vi "Configure Function.vi"(0 "VISA resource name":refnum<visa-resource-name>, 1 "Channel":i8 min=0 max=20 step=1, 5 "Function (5: Temp)":u16(ring)=5 items=["OFF", "VDC", "VAC", "OHMS", "FREQ", "TEMP"], 7 "Thermocouple Type (0: J) 2":u16(ring)=5 items=["J", "K", "E", "T", "N", "R", "S", "B", "C"], 9 "Frequency (0: 900 Hz)":u16(ring)=5 items=["900 Hz", "9 kHz", "90 kHz", "900 kHz", "1 MHz"], 11 "error in (no error)":errorcluster, 12 "Resistance (0: 300 Ohms)  2":u16(ring)=5 items=["300 Ohms", "3 k Ohms", "30 k Ohms", "300 k Ohms", "3 M Ohms", "10 M Ohms"], 13 "Voltage (0: 300 mV)  3":u16(ring)=5 items=["300 mV", "3 V", "30 V", "150/300 V", "3 M Ohms", "10 M Ohms"]) -> (4 "VISA resource name out":refnum<visa-resource-name>, 6 "concatenated string":string, 10 "read buffer":string, 15 "error out":errorcluster)   [LabVIEW 2013]
doc: "Configures the measurement type, resolution, and range on the instrument."
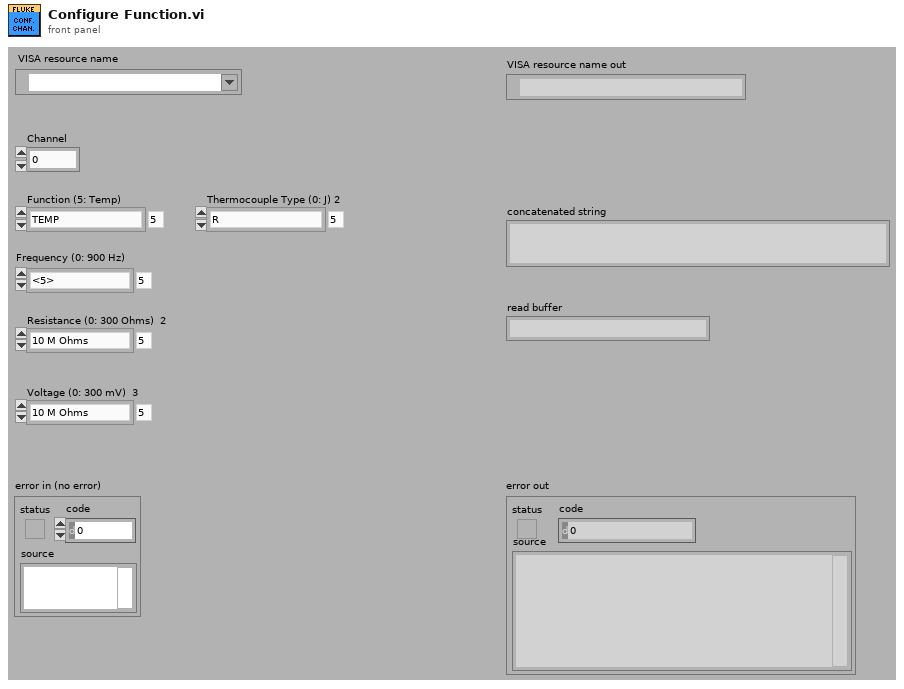
[diagram p1: front panel]
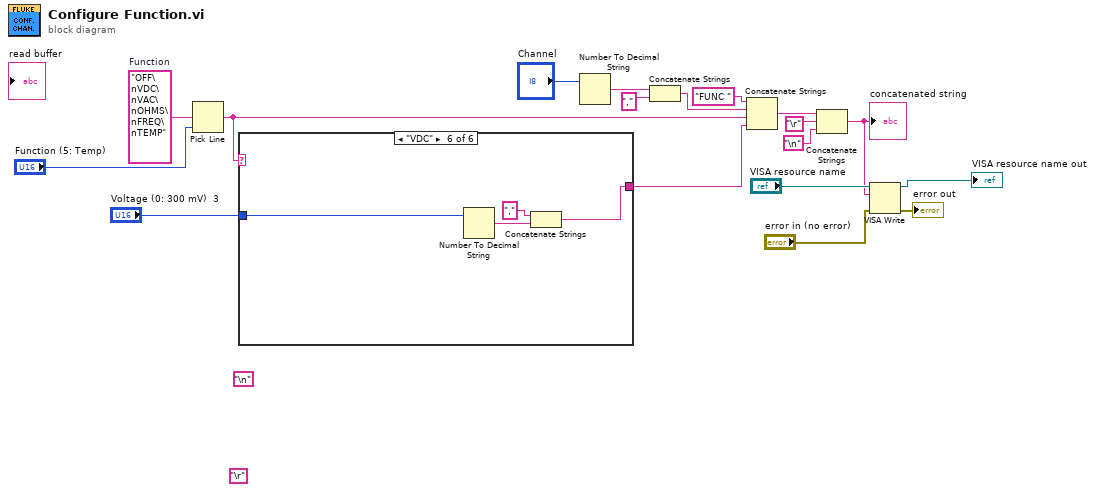
[diagram p0: block diagram]
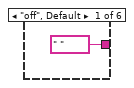
[diagram p2: hidden frame]
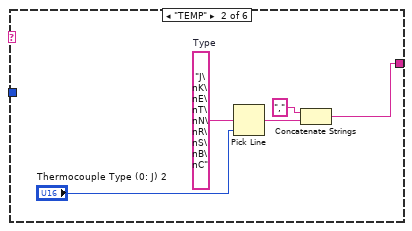
[diagram p3: hidden frame]
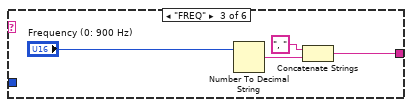
[diagram p4: hidden frame]
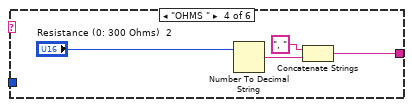
[diagram p5: hidden frame]
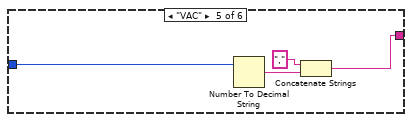
[diagram p6: hidden frame]
diagram:
  w18 = "OFF\nVDC\nVAC\nOHMS\nFREQ\nTEMP"  # Function
  (unwired) "\n"
  (unwired) "\r"
  n1 = Pick Line(multi-line string=w18, line index="Function (5: Temp)") -> (output string=w10:string)  [unwired: 1 in]
  n2 = case shown="\"VDC\"" w10 {
    tunnel: [" " w24 w27 w31 w33 w39] -> w11
    tunnel: "Voltage (0: 300 mV)  3" -> [_ _ _ _ w36 w40]
    frame "off", Default {
    }
    frame "TEMP" {
      w23 = "J\nK\nE\nT\nN\nR\nS\nB\nC"  # Type
      n3 = Pick Line(multi-line string=w23, line index="Thermocouple Type (0: J) 2") -> (output string=w21:string)  [unwired: 1 in]
      n4 = Concatenate Strings("," ("string"), w21) -> (w24:string)
    }
    frame "FREQ" {
      n5 = Number To Decimal String(number="Frequency (0: 900 Hz)") -> (decimal integer string=w25:string)  [unwired: 1 in]
      n6 = Concatenate Strings(", ", w25) -> (w27:string)
    }
    frame "OHMS " {
      n7 = Number To Decimal String(number="Resistance (0: 300 Ohms)  2") -> (decimal integer string=w29:string)  [unwired: 1 in]
      n8 = Concatenate Strings(", ", w29) -> (w31:string)
    }
    frame "VAC" {
      n9 = Number To Decimal String(number=w36) -> (decimal integer string=w34:string)  [unwired: 1 in]
      n10 = Concatenate Strings(",", w34) -> (w33:string)
    }
    frame "VDC" {
      n11 = Number To Decimal String(number=w40) -> (decimal integer string=w37:string)  [unwired: 1 in]
      n12 = Concatenate Strings(",", w37) -> (w39:string)
    }
  }
  n13 = Number To Decimal String(number="Channel") -> (decimal integer string=w14:string)  [unwired: 1 in]
  n14 = Concatenate Strings(w14, ",") -> (w12:string)
  n15 = Concatenate Strings("FUNC ", w12, w10, w11) -> (w6:string)
  n16 = Concatenate Strings(w6, "\r", "\n") -> (w2:string)
  "concatenated string" <- w2
  n17 = VISA Write(VISA resource name="VISA resource name", write buffer=w2, error in (no error)="error in (no error)") -> (VISA resource name out=→"VISA resource name out":refnum<visa-resource-name>, error out=→"error out":errorcluster)  [unwired: 1 out]
